vi "Joystick Get.vi"(11 "Js name":string) -> (0 "axis 4":dbl, 1 "axis 3 (throttle)":dbl, 2 "axis 2 (y)":dbl, 3 "axis 1 (x)":dbl, 4 "Button 12":bool, 5 "Button 1":bool)   [LabVIEW 2012]
uses:
  <vilib>/Rock Robotics/WPI/Joystick/WPI_JoystickGetSetRefNum.vi
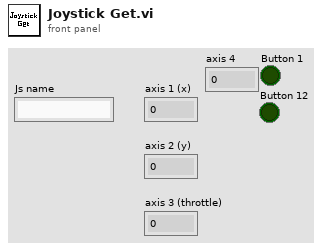
[diagram p1: front panel]
types:
  T1 = typedef "WPI_JoystickDevRef.ctl" = cluster{"Device":T2}
  T2 = typedef "WPI_JoystickDeviceEnum.ctl" = enum16{"USB 1", "USB 2", "USB 3", "USB 4", "Kinect 1", "Kinect 2"}
  T3 = typedef "WPI_JoystickButtonState.ctl" = cluster{"Button 1":bool, "Button 2":bool, "Button 3":bool, "Button 4":bool, "Button 5":bool, "Button 6":bool, "Button 7":bool, "Button 8":bool, "Button 9":bool, "Button 10":bool, "Button 11":bool, "Button 12":bool}
  T4 = cluster{"axis 1 (x)":dbl, "axis 2 (y)":dbl, "axis 3 (throttle)":dbl, "axis 4":dbl, "axis 5":dbl, "axis 6":dbl}
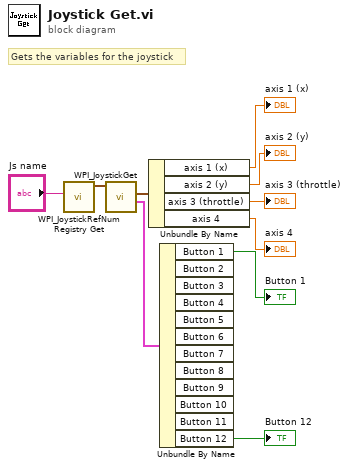
[diagram p0: block diagram]
diagram:
  # "Gets the variables for the joystick"
  n1 = call <vilib>:"WPI_JoystickRefNum Registry Get.vi"("refnum name"="Js name") -> ("JoystickDevRef"=w6:T1)  [unwired: 9 in, 1 out]
  n2 = call <vilib>:"WPI_JoystickGet.vi"("JoystickDevRef"=w6) -> ("Buttons"=w3:T3, "Axes"=w7:T4)  [unwired: 4 in, 1 out]
  n3 = Unbundle By Name(w7) -> ("axis 1 (x)"=→"axis 1 (x)":dbl, "axis 2 (y)"=→"axis 2 (y)":dbl, "axis 3 (throttle)"=→"axis 3 (throttle)":dbl, "axis 4"=→"axis 4":dbl)
  n4 = Unbundle By Name(w3) -> ("Button 1"=→"Button 1":bool, "Button 12"=→"Button 12":bool)  [unwired: 10 out]
